vi "Autonomous_Routine_Global.vi"() -> ()   [LabVIEW 2012]
panel:
  in  "Reset":bool
  in  "CamPidOn":bool
  in  "Cam Setpoint":dbl
  in  "FIRE":bool
  in  "FireTime(ms)":dbl=1000.0
  in  "UpdatingCurrentCamPosition":dbl
  in  "PreviousCamPosition":dbl
  in  "Is The Cannon In An Autonomous Routine?":bool
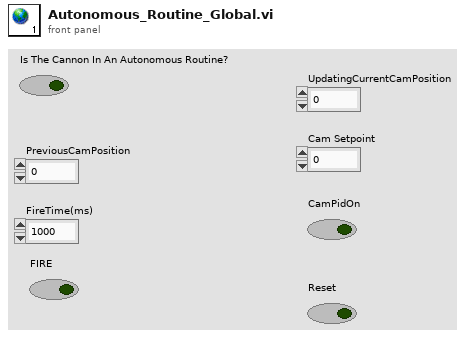
[diagram p1: front panel]
diagram:
